vi "ReversedEngineering GetDiagramStateMachineInfo.vi"(1 "Path":path=path "C:/Documents and Settings/MikaelH/My Documents/LabView/StateMachine-JKI/StateMachine3.vi", 2 "StateDiagramReverseOptions":T1={"Clear All Current States"=TRUE, "UseMenuItem"=TRUE, "InsertArrayQueuedElementsVI"="", "Add Actions"=TRUE, "StateDiagramSerachActions"={"Action"=enum."OnlyTheseVIs", "VINames"=[], "LimitActions(VIs)"=0}, "AddCaseCommentsAsActions"=FALSE, "IgnoreStatesNotUsed"=FALSE, "CommentsSerachActions"={"MinimumTextLength"=0, "OnlyTopLeftComment"=FALSE, "CommentPrefix"=""}, "TransitionMode"=enum."Add to current transtion text", "ActionMode"=enum."Add to current action text"}, 5 "error in (no error)":errorcluster) -> (15 "States":T5[](array[typedef]), 19 "error out":errorcluster)   [LabVIEW 2014]
uses:
  <resource>/Framework/Providers/Open_GDS/UML/ReversedEngineering/ReversedEngineering StateMachineStateInfo.ctl
  <resource>/Framework/Providers/Open_GDS/UML/ReversedEngineering/private/ReversedEngineering StateDiagramReverseOptions.ctl
  <resource>/Framework/Providers/Open_GDS/UML/ReversedEngineering/private/ReversedEngineering StateDiagramSerachActions.ctl
  <resource>/Framework/Providers/Open_GDS/UML/ReversedEngineering/ReversedEngineering StateAnalyseVIAction.ctl
  <resource>/Framework/Providers/Open_GDS/UML/ReversedEngineering/private/ReversedEngineering StateDiagramCommentSearchType.ctl
  <resource>/Framework/Providers/Open_GDS/UML/StateReverse_class/StateAction.ctl
  <resource>/Framework/Providers/Open_GDS/UML/ReversedEngineering/ReversedEngineering QueuedStateMachinMemoryAction.ctl
  <resource>/Framework/Providers/Open_GDS/UML/UMLEditor/UMLEditor BusyDialogAction.ctl
  <resource>/Framework/Providers/Open_GDS/ClassProviders/Common/ScriptingFunctions/Scripting.lvclass
  <resource>/Framework/Providers/Open_GDS/UML/StateReverse_class/StateReverse.lvclass
panel:
  out "StateTransitions":cluster{"StateTransitions":string[]}[](array[cluster])
  out "SubViNames":string[](array[string])
  out "Selector Strings":string[](array[string])
  # "C:\\Documents and Settings\\Micke\\Mina dokument\\LabView\\StateMachines\\String1\\StateString1.vi"
  # "C:\\Documents and Settings\\MikaelH\\My Documents\\LabView\\StateMachine-JKI\\StateMachine3.vi"
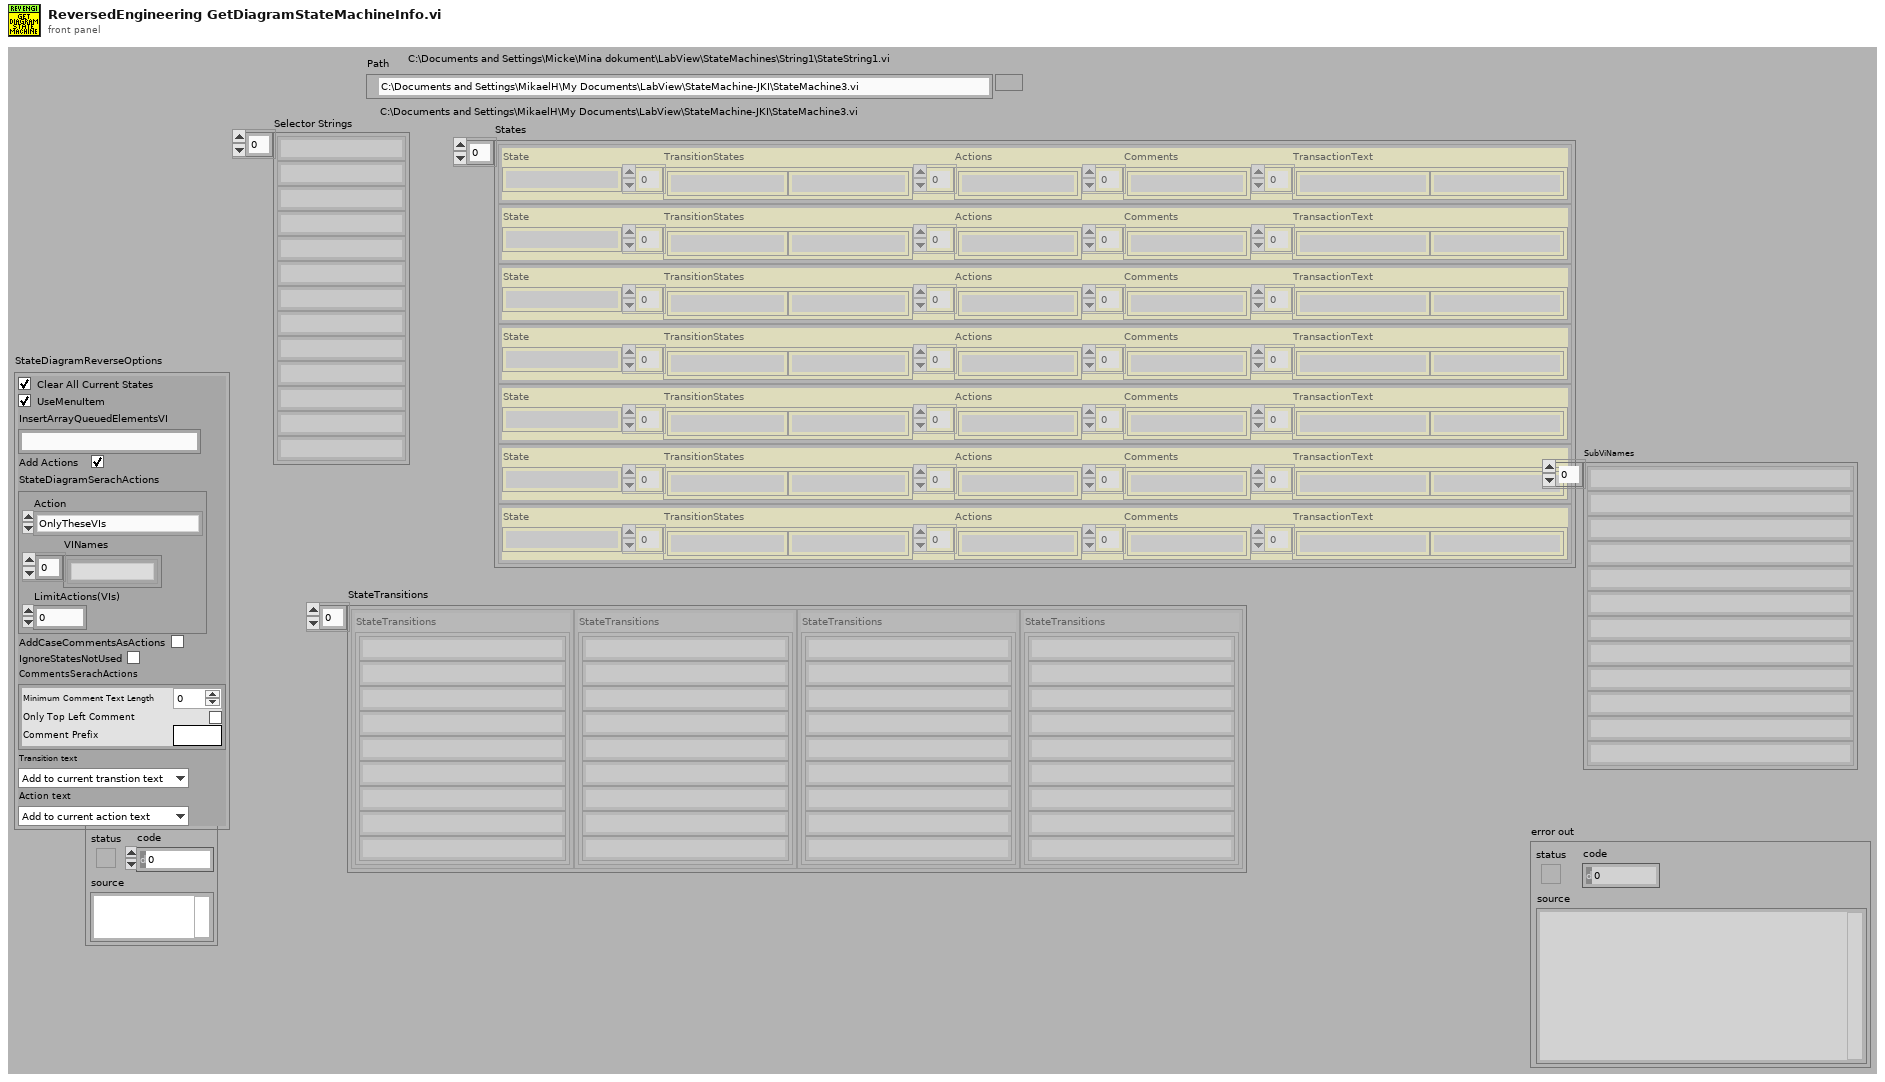
[diagram p1: front panel]
types:
  T1 = typedef "ReversedEngineering StateDiagramReverseOptions.ctl" = cluster{"Clear All Current States":bool, "UseMenuItem":bool, "InsertArrayQueuedElementsVI":string, "Add Actions":bool, "StateDiagramSerachActions":T2, "AddCaseCommentsAsActions":bool, "IgnoreStatesNotUsed":bool, "CommentsSerachActions":T4, "TransitionMode":enum16{"Add to current transtion text", "Replace transition text"}, "ActionMode":enum16{"Add to current action text", "Replace action text"}}
  T2 = typedef "ReversedEngineering StateDiagramSerachActions.ctl" = cluster{"Action":T3, "VINames":string[], "LimitActions(VIs)":i32}
  T3 = typedef "ReversedEngineering StateAnalyseVIAction.ctl" = enum16{"OnlyTheseVIs", "NotTheseVIs"}
  T4 = typedef "ReversedEngineering StateDiagramCommentSearchType.ctl" = cluster{"MinimumTextLength":i32, "OnlyTopLeftComment":bool, "CommentPrefix":string}
  T5 = typedef "ReversedEngineering StateMachineStateInfo.ctl" = cluster{"State":string, "TransitionStates":string[], "Actions":string[], "Comments":string[], "TransactionText":string[]}
  T6 = typedef "Scripting.lvclass/Scripting_PastThroughObjectType.ctl" = cluster{"Object":refnum<vi>, "InsideArray":bool, "PastThroughObjectTypes":T7[], "ObjectType":string, "ObjectData":string}
  T7 = typedef "Scripting_ObjectType.ctl" = cluster{"ObjectType":string, "ObjectName":string, "ObjectTerminalName":string}
  T8 = typedef "StateReverse.lvclass/StateAction.ctl" = enum16{"Normal", "AddInBeggining", "AddInEnd", "AddIfNothingInQueue"}
  T9 = enum16{"NormalSubVis", "LV-Internal VIs", "All VIs", "All Functions"}
  T10 = typedef "ReversedEngineering QueuedStateMachinMemoryAction.ctl" = enum16{"Initialize", "GetInsertQueuedArrayElementsVI", "SetQueuedStateJumps", "GetQueuedStateJumps"}
  T11 = typedef "UMLEditor BusyDialogAction.ctl" = enum16{"Initialize", "Open(VIs)", "Open(i)", "Send_I-Value", "SendStatusMessage", "GetBusyDialogStatus", "Close", "Quit"}
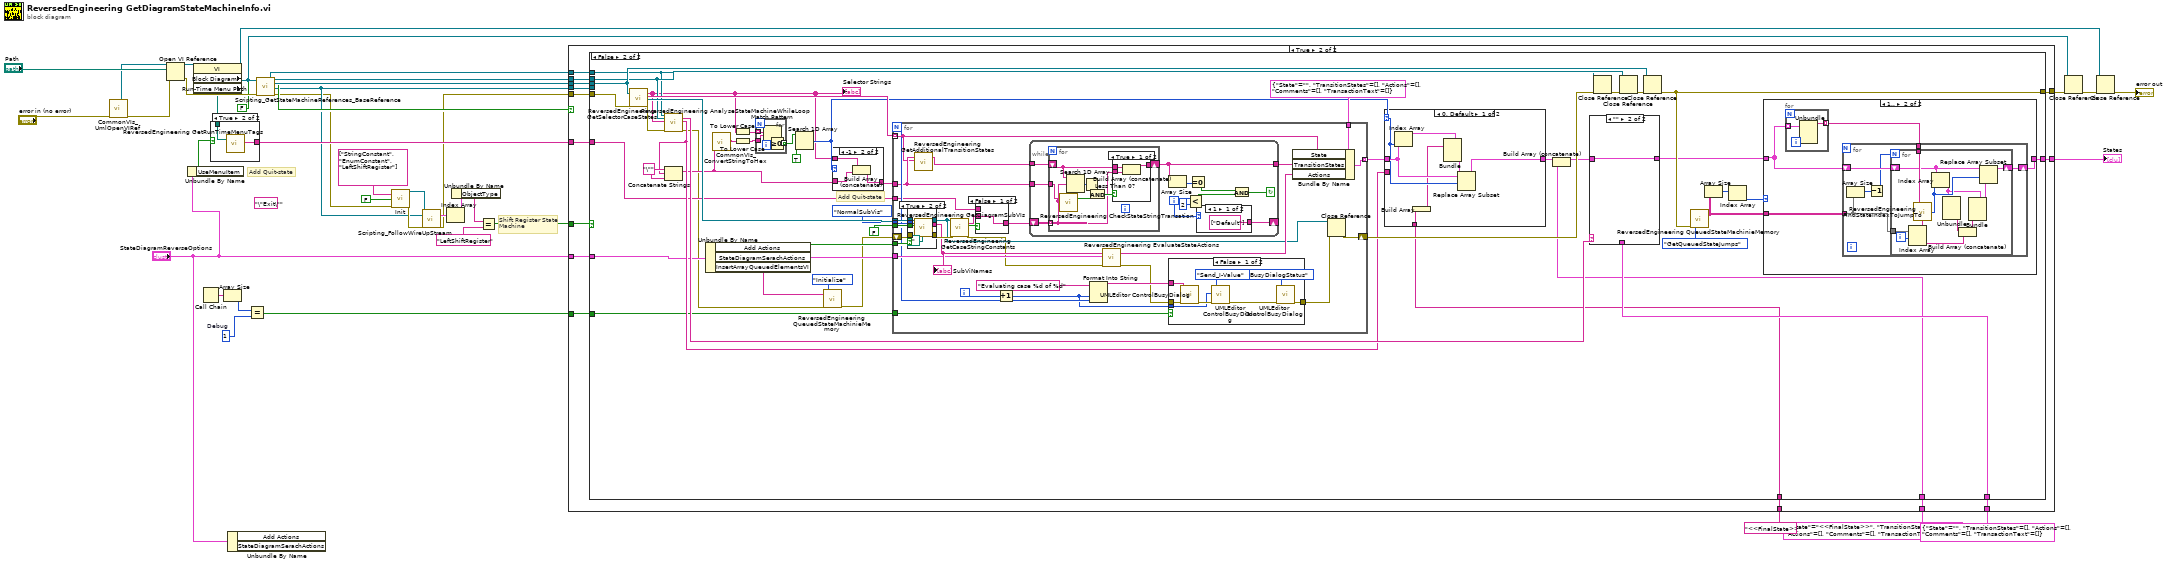
[diagram p0: block diagram]
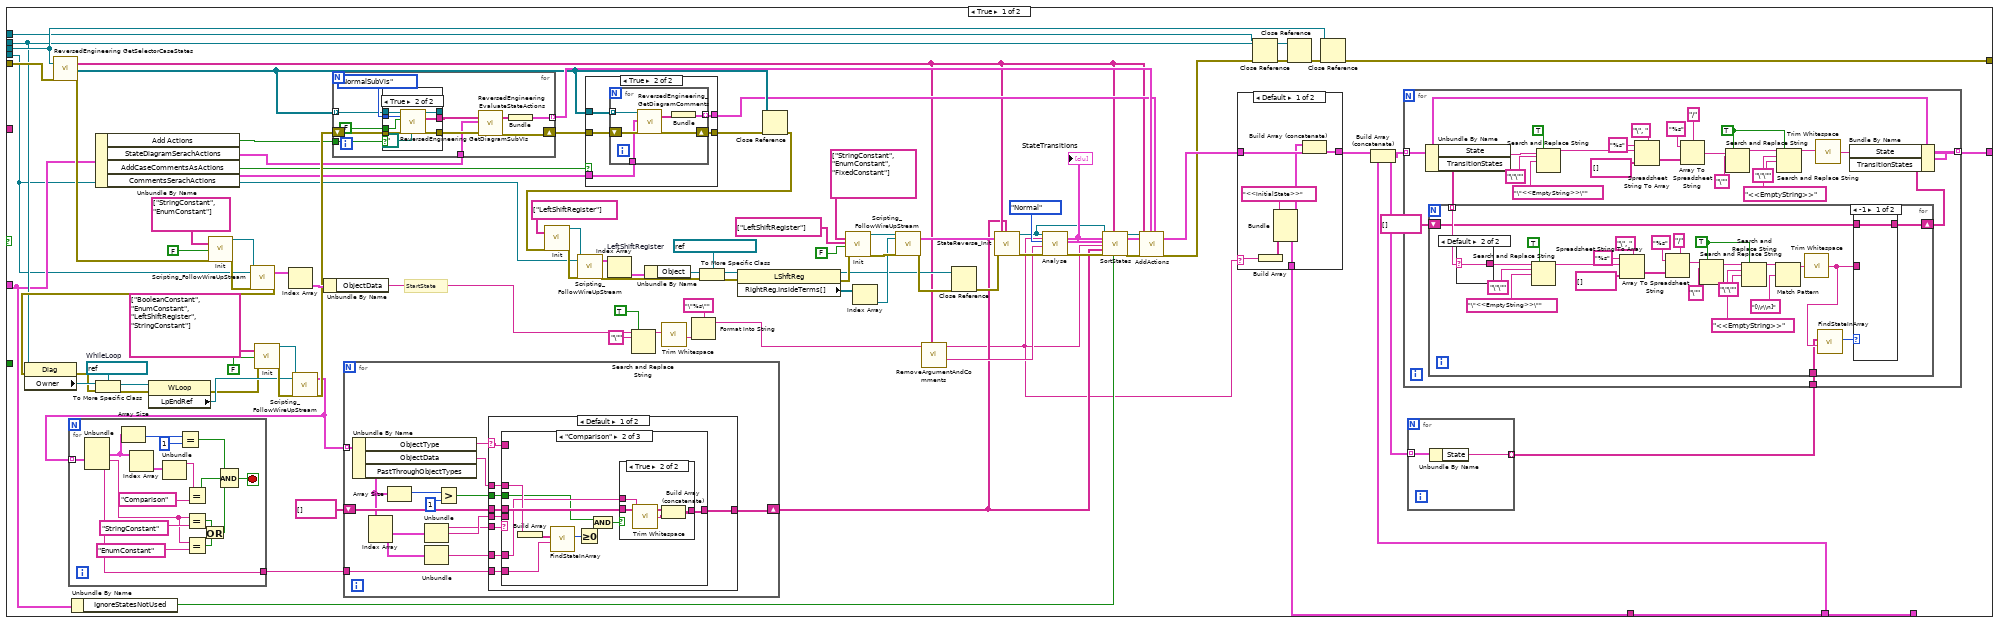
[diagram p4: hidden frame]
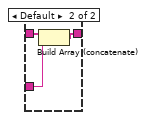
[diagram p7: hidden frame]
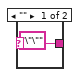
[diagram p8: hidden frame]
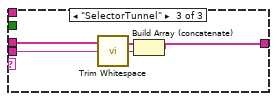
[diagram p11: hidden frame]
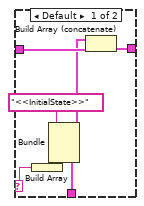
[diagram p15: hidden frame]
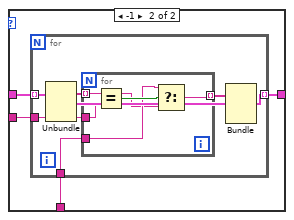
[diagram p16: hidden frame]
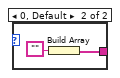
[diagram p18: hidden frame]
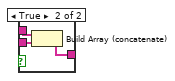
[diagram p20: hidden frame]
diagram:
  w24 = 1  # Debug
  (unwired) "\"Exit\"" ("element")
  # "Shift Register State\nMachine"
  # "Add Quit-state"
  n1 = call <resource>:"CommonVIs_UmlOpenVIRef.vi"("error in"="error in (no error)") -> ("error out"=w2:errorcluster, "AppRefOut"=w1:refnum<vi>)  [unwired: 3 in, 6 out]
  n2 = Open VI Reference(application reference (local)=w1, vi path="Path", error in (no error)=w2) -> (vi reference=w22:refnum<vi>, error out=w39:errorcluster)  [unwired: 3 out]
  n3 = Unbundle By Name("StateDiagramReverseOptions") -> ("UseMenuItem"=w19:bool)
  n4 = property class="VI"(reference=w22) -> (reference out=w32:refnum<vi>, "Block Diagram"=w21:refnum<vi>, "Run-Time Menu Path"=w20:path)  [unwired: 1 in, 1 out]
  n5 = Call Chain() -> (call chain=w26:string[])
  n6 = case shown="True" w19 {
    tunnel: w20 -> [_ w42]
    tunnel: [_ w41] -> w18
    frame False {
    }
    frame True {
      n7 = call <resource>:"ReversedEngineering GetRunTimeMenuTags.vi"("StateMachineCaseSelector"=w42) -> ("ItemTags"=w41:string[])  [unwired: 1 in, 17 out]
    }
  }
  n8 = Array Size(array=w26) -> (size(s)=w25:i32)
  n9 = Unbundle By Name("StateDiagramReverseOptions") -> ()  [unwired: 2 out]
  n10 = Equal?(x=w25, y=w24) -> (x = y?=w23:bool)
  n11 = call <resource>:"Scripting_GetStateMachineReferences_BaseReference.vi"("Diagram"=w21, "WhileLoop(False)"=FALSE, "error in (no error)"=w39) -> ("OutSideWhileLoopDiagram"=w34:refnum<vi>, "StateMachine-WhileLoopDiagram"=w35:refnum<vi>, "StateMachine-CaseSelector"=w38:refnum<vi>, "Found"=w37:bool, "Selector.Outside Terminal"=w12:refnum<vi>, "error out"=w6:errorcluster)  [unwired: 11 in]
  n12 = call <resource>:"Init.vi"("FindAnyOfTheseClassTypes"=string[] ["StringConstant", "EnumConstant", "LeftShiftRegister"], "KeepObjectsOpen(True)"=FALSE, "error in (no error)"=w6) -> ("object out"=w13:refnum<class "Scripting.lvclass">, "error out"=w14:errorcluster)  [unwired: 15 in]
  n13 = call-dynamic "Scripting_FollowWireUpStream.vi"("Scripting in"=w13, "StartTerminalRef"=w12, "error in (no error)"=w14) -> ("FoundItems"=w11:T6[], "error out"=w5:errorcluster)  [unwired: 15 in]
  n14 = Index Array(array=w11) -> (element=w10:T6)  [unwired: 1 in]
  n15 = Unbundle By Name(w10) -> ("ObjectType"=w9:string)
  n16 = Equal?(x=w9, y="LeftShiftRegister" ("StopWhenThisClassTypeReached")) -> (x = y?=w7:bool)
  n17 = case shown="True" w37 {
    tunnel: w38 -> [_ w57]
    tunnel: w5 -> [w43 w50]
    tunnel: [w43 w47] -> w31
    tunnel: [_ w46] -> w36
    tunnel: w35 -> [_ w56]
    tunnel: w34 -> [_ w55]
    tunnel: T5 {"State"="", "TransitionStates"=[], "Actions"=[], "Comments"=[], "TransactionText"=[]} ("State") -> [_ w54]
    tunnel: T5 {"State"="<<FinalState>>", "TransitionStates"=[], "Actions"=[], "Comments"=[], "TransactionText"=[]} ("State") -> [_ w52]
    tunnel: "<<FinalState>>" ("State") -> [_ w53]
    tunnel: "StateDiagramReverseOptions" -> [_ w51]
    tunnel: w23 -> [_ w49]
    tunnel: w18 -> [_ w48]
    tunnel: w12 -> [_ w45]
    tunnel: w7 -> [_ w44]
    frame False {
    }
    frame True {
      n18 = case shown="False" w44 {
        tunnel: w57 -> [w150 w354]
        tunnel: w56 -> [w124 w351]
        tunnel: w55 -> [w148 w350]
        tunnel: w54 -> [w147 w348]
        tunnel: w53 -> [_ w346]
        tunnel: w52 -> [w88 w344]
        tunnel: w51 -> [w73 w339]
        tunnel: w50 -> [w145 w329]
        tunnel: w49 -> [_ w325]
        tunnel: w48 -> [_ w324]
        tunnel: [w144 w319] -> w47
        tunnel: [w90 w314] -> w46
        tunnel: w45 -> [w71 _]
        frame True {
          w118 = refnum<vi> refnum  # LeftShiftRegister
          w143 = refnum<vi> refnum  # WhileLoop
          # "StartState"
          n19 = call <resource>:"ReversedEngineering GetSelectorCaseStates.vi"("StateMachineCaseSelector"=w150, "error out 2"=w145) -> ("SelStrings"=w63:string[], "Frames[]"=w76:refnum<vi>[], "error out"=w126:errorcluster)  [unwired: 2 in, 13 out]
          n20 = Unbundle By Name(w73) -> ("IgnoreStatesNotUsed"=w72:bool)
          n21 = Unbundle By Name(w73) -> ("Add Actions"=w86:bool, "StateDiagramSerachActions"=w85:T2, "AddCaseCommentsAsActions"=w78:bool, "CommentsSerachActions"=w70:T4)
          n22 = call <resource>:"Init.vi"("FindAnyOfTheseClassTypes"=string[] ["StringConstant", "EnumConstant"], "KeepObjectsOpen(True)"=FALSE, "error in (no error)"=w126) -> ("object out"=w131:refnum<class "Scripting.lvclass">, "error out"=w130:errorcluster)  [unwired: 15 in]
          n23 = call-dynamic "Scripting_FollowWireUpStream.vi"("Scripting in"=w131, "StartTerminalRef"=w71, "error in (no error)"=w130) -> ("FoundItems"=w132:T6[], "error out"=w125:errorcluster)  [unwired: 15 in]
          n24 = property class="Diag"(reference=w124, error in=w125) -> (error out=w133:errorcluster, "Owner"=w134:refnum<vi>)  [unwired: 1 out]
          n25 = To More Specific Class(target class=w143, reference=w134, error in=w133) -> (specific class reference=w142:refnum<vi>, error out=w137:errorcluster)
          n26 = property class="WLoop"(reference=w142, error in=w137) -> (error out=w138:errorcluster, "LpEndRef"=w139:refnum<vi>)  [unwired: 1 out]
          n27 = call <resource>:"Init.vi"("FindAnyOfTheseClassTypes"=string[] ["BooleanConstant", "EnumConstant", "LeftShiftRegister", "StringConstant"], "KeepObjectsOpen(True)"=FALSE, "error in (no error)"=w138) -> ("object out"=w140:refnum<class "Scripting.lvclass">, "error out"=w141:errorcluster)  [unwired: 15 in]
          n28 = Index Array(array=w132) -> (element=w127:T6)  [unwired: 1 in]
          n29 = call-dynamic "Scripting_FollowWireUpStream.vi"("Scripting in"=w140, "StartTerminalRef"=w139, "error in (no error)"=w141) -> ("FoundItems"=w59:T6[], "error out"=w87:errorcluster)  [unwired: 15 in]
          n30 = for {
            tunnel: w59 -> [w167] mode=indexing
            tunnel: [w151] -> w58
            stop <- w152 stop-if-true
            n31 = Unbundle(w167) -> ("PastThroughObjectTypes"=w163:T7[], "ObjectType"=w159:string, "ObjectData"=w151:string)  [unwired: 2 out]
            n32 = Array Size(array=w163) -> (size(s)=w162:i32)
            n33 = Index Array(array=w163) -> (element=w164:T7)  [unwired: 1 in]
            n34 = Unbundle(w164) -> ("ObjectType"=w166:string)  [unwired: 2 out]
            n35 = Equal?(x=w162, y=1) -> (x = y?=w155:bool)
            n36 = Equal?(x=w166, y="Comparison") -> (x = y?=w154:bool)
            n37 = Equal?(x=w159, y="StringConstant" ("StopWhenThisClassTypeReached")) -> (x = y?=w157:bool)
            n38 = Equal?(x=w159, y="EnumConstant" ("StopWhenThisClassTypeReached")) -> (x = y?=w156:bool)
            n39 = Or(x=w157, y=w156) -> (x .or. y?=w153:bool)
            n40 = Compound Arithmetic op=AND(w155, w154, w153) -> (w152:bool)
          }
          n41 = Unbundle By Name(w127) -> ("ObjectData"=w91:string)
          n42 = for {
            tunnel: w86 -> [w192]
            shift-right: [w187] -> w79
            shift-left: w87 -> [w190]
            tunnel: w85 -> [w185]
            tunnel: w76 -> [w184] mode=indexing
            tunnel: [w182] -> w80 mode=indexing
            n43 = case shown="True" w192 {
              tunnel: [w193 w202] -> _
              tunnel: w190 -> [w194 w201]
              tunnel: [w194 w200] -> w191
              tunnel: T9."NormalSubVis" ("SubVIsOptions(NormalSubVis)") -> [_ w199]
              tunnel: [_ w198] -> w186
              tunnel: FALSE ("RecrsiveSearchInNormalSubVIs(False)") -> [_ w197]
              tunnel: w184 -> [w193 w196]
              frame False {
              }
              frame True {
                n44 = call <resource>:"ReversedEngineering GetDiagramSubVIs.vi"("Diagram"=w196, "SubVIsOptions(NormalSubVis)"=w199, "RecrsiveSearchInNormalSubVIs(False)"=w197, "error in (no error)"=w201, "PathToDebugVI(OnlyUsedForRecursivVitFiles)"=path "") -> ("DiagramOut"=w202:refnum<vi>, "SubViNames"=w198:string[], "error out"=w200:errorcluster)  [unwired: 12 out]
              }
            }
            n45 = call <resource>:"ReversedEngineering EvaluateStateActions.vi"("SubViNames"=w186, "StateDiagramSerachActions"=w185, "error in"=w191) -> ("StateActions"=w183:string[], "error out"=w187:errorcluster)  [unwired: 15 out]
            n46 = Bundle("StateActions"=w183) -> (w182:cluster{"StateActions":string[]})  [unwired: 1 in]
          }
          n47 = for {
            tunnel: w59 -> [w274] mode=indexing
            shift-right: [w271] -> w62
            shift-left: string[] [] -> [w272]
            tunnel: w58 -> [w264]
            n48 = Unbundle By Name(w274) -> ("ObjectType"=w273:string, "ObjectData"=w268:string, "PastThroughObjectTypes"=w261:T7[])
            n49 = Index Array(array=w261) -> (element #1=w267:T7, element #2=w266:T7)  [unwired: 2 in]
            n50 = Array Size(array=w261) -> (size(s)=w263:i32)
            n51 = Unbundle(w267) -> ("ObjectType"=w269:string, "ObjectName"=w270:string)  [unwired: 1 out]
            n52 = Unbundle(w266) -> ("ObjectName"=w265:string)  [unwired: 2 out]
            n53 = Greater?(x=w263, y=1) -> (0:w260:bool)
            n54 = case shown="Default" w273 {
              selector: w273 -> [w279 _]
              tunnel: w272 -> [w283 w304]
              tunnel: [w282 w304] -> w271
              tunnel: w270 -> [w281 _]
              tunnel: w269 -> [w280 _]
              tunnel: w268 -> [w278 _]
              tunnel: w265 -> [w277 _]
              tunnel: w264 -> [w276 _]
              tunnel: w260 -> [w275 _]
              frame Default {
                n55 = case shown="\"Comparison\"" w280 {
                  tunnel: w283 -> [w284 w294 w303]
                  tunnel: [w284 w293 w302] -> w282
                  tunnel: w281 -> [_ _ w301]
                  tunnel: w279 -> [_ _ _]
                  tunnel: w278 -> [_ w289 _]
                  tunnel: w277 -> [_ w288 _]
                  tunnel: w276 -> [_ w290 _]
                  tunnel: w275 -> [_ w285 _]
                  frame Default {
                  }
                  frame "Comparison" {
                    n56 = Build Array(w289) -> (w291:string[])
                    n57 = call <resource>:"FindStateInArray.vi"("TransactionState"=w290, "AllCaseStates"=w291) -> ("index of element"=w292:i32)  [unwired: 7 in, 2 out]
                    n58 = Greater Or Equal To 0?(x=w292) -> (x >= 0?=w287:bool)
                    n59 = And(x=w285, y=w287) -> (x .and. y?=w286:bool)
                    n60 = case shown="True" w286 {
                      tunnel: w294 -> [w295 w298]
                      tunnel: [w295 w297] -> w293
                      tunnel: w288 -> [_ w296]
                      frame False {
                      }
                      frame True {
                        n61 = call <vilib>:"Trim Whitespace.vi"("string"=w296) -> ("trimmed string"=w299:string)  [unwired: 1 in]
                        n62 = Build Array (concatenate)(w298, w299) -> (w297:string[])
                      }
                    }
                  }
                  frame "SelectorTunnel" {
                    n63 = call <vilib>:"Trim Whitespace.vi"("string"=w301) -> ("trimmed string"=w300:string)  [unwired: 1 in]
                    n64 = Build Array (concatenate)(w303, w300) -> (w302:string[])
                  }
                }
              }
              frame "UseDefault" {
              }
            }
          }
          n65 = case shown="True" w78 {
            tunnel: w79 -> [w170 w175]
            tunnel: w76 -> [_ w174]
            tunnel: [w170 w173] -> w77
            tunnel: [_ w172] -> w75
            tunnel: w70 -> [_ w171]
            frame False {
            }
            frame True {
              n66 = for {
                tunnel: w174 -> [w180] mode=indexing
                shift-right: [w179] -> w173
                shift-left: w175 -> [w181]
                tunnel: [w177] -> w172 mode=indexing
                tunnel: w171 -> [w176]
                n67 = call <resource>:"ReversedEngineering_GetDiagramComments.vi"("Diagram"=w180, "CommentsSerachActions"=w176, "error in"=w181) -> ("Comments"=w178:string[], "error out"=w179:errorcluster)  [unwired: 15 in]
                n68 = Bundle("Comments"=w178) -> (w177:cluster{"Comments":string[]})  [unwired: 1 in]
              }
            }
          }
          n69 = Search and Replace String(replace all?=TRUE ("replace all? (F)"), input string=w91, search string="\"") -> (result string=w94:string)  [unwired: 5 in, 3 out]
          n70 = call <vilib>:"Trim Whitespace.vi"("string"=w94) -> ("trimmed string"=w92:string)  [unwired: 1 in]
          n71 = Format Into String(format string="\"%s\"", w92) -> (resulting string=w65:string)  [unwired: 2 in, 1 out]
          n72 = Close Reference(reference=w76, error in (no error)=w77) -> (error out=w74:errorcluster)
          n73 = call <resource>:"Init.vi"("FindAnyOfTheseClassTypes"=string[] ["LeftShiftRegister"], "error in (no error)"=w74) -> ("object out"=w122:refnum<class "Scripting.lvclass">, "error out"=w123:errorcluster)  [unwired: 16 in]
          n74 = call-dynamic "Scripting_FollowWireUpStream.vi"("Scripting in"=w122, "StartTerminalRef"=w71, "error in (no error)"=w123) -> ("FoundItems"=w121:T6[], "error out"=w117:errorcluster)  [unwired: 15 in]
          n75 = Index Array(array=w121) -> (element=w120:T6)  [unwired: 1 in]
          n76 = Unbundle By Name(w120) -> ("Object"=w119:refnum<vi>)
          n77 = To More Specific Class(target class=w118, reference=w119, error in=w117) -> (specific class reference=w116:refnum<vi>, error out=w115:errorcluster)
          n78 = property class="LShftReg"(reference=w116, error in=w115) -> (reference out=w104:refnum<vi>, error out=w109:errorcluster, "RightReg.InsideTerms[]"=w114:refnum<vi>[])
          n79 = call <resource>:"Init.vi"("FindAnyOfTheseClassTypes"=string[] ["StringConstant", "EnumConstant", "FixedConstant"], "StopWhenAnyOfTheseClassTypesAreReached"=string[] ["LeftShiftRegister"] ("FindAnyOfTheseClassTypes"), "KeepObjectsOpen(True)"=FALSE, "error in (no error)"=w109) -> ("object out"=w111:refnum<class "Scripting.lvclass">, "error out"=w113:errorcluster)  [unwired: 14 in]
          n80 = Index Array(array=w114) -> (element=w110:refnum<vi>)  [unwired: 1 in]
          n81 = call-dynamic "Scripting_FollowWireUpStream.vi"("Scripting in"=w111, "StartTerminalRef"=w110, "error in (no error)"=w113) -> ("FoundItems"=w100:T6[], "error out"=w105:errorcluster)  [unwired: 15 in]
          n82 = call <resource>:"RemoveArgumentAndComments.vi"("AllCaseStates"=w63, "TransactionStateIn"=w65) -> ("Comment"=w64:string, "TransactionStateOut"=w61:string)  [unwired: 7 in, 1 out]
          n83 = Close Reference(reference=w104, error in (no error)=w105) -> (error out=w101:errorcluster)
          n84 = call <resource>:"StateReverse_Init.vi"("StatesData"=w100, "error in (no error)"=w101, "StateStrings"=w63, "ExitStates"=w62) -> ("object out"=w67:refnum<class "StateReverse.lvclass">, "error out"=w103:errorcluster)  [unwired: 14 in]
          n85 = call-dynamic "Analyse.vi"("object in"=w67, "NextState"=w61, "StateAction"=StateAction."Normal", "NextStateComments"=w64, "error in (no error)"=w103) -> ("StateTransitions"=w98:cluster{"StateTransitions":string[]}[], "CommentsTransitions"=w60:cluster{"StateTransitions":string[]}[], "error out"=w97:errorcluster)  [unwired: 12 in]
          "StateTransitions" <- w98
          n86 = call <resource>:"SortStates.vi"("object in"=w67, "StateTransitions"=w98, "CommentsTransitions"=w60, "StartState"=w61, "ExitStates"=w62, "error in (no error)"=w97, "StateStrings"=w63, "RemoveStatesNotInUse(True)"=w72) -> ("object out"=w66:refnum<class "StateReverse.lvclass">, "States"=w84:T5[], "error out"=w83:errorcluster)  [unwired: 9 in]
          n87 = call <resource>:"AddActions.vi"("object in"=w66, "StatesIn"=w84, "error in (no error)"=w83, "StateStrings"=w63, "StateActions"=w80, "StateComments"=w75) -> ("States"=w82:T5[], "error out"=w81:errorcluster)  [unwired: 11 in, 1 out]
          n88 = case shown="Default" w61 {
            selector: w61 -> [w307 _]
            tunnel: w82 -> [w311 w312]
            tunnel: [w310 w312] -> w89
            tunnel: w147 -> [w309 _]
            frame Default {
              n89 = Build Array(w307) -> (w306:string[])
              n90 = Bundle(cluster=w309, "State"="<<InitialState>>", "TransitionStates"=w306) -> (w305:T5)  [unwired: 3 out]
              n91 = Build Array (concatenate)(w305, w311) -> (w310:T5[])
            }
            frame "" {
            }
          }
          n92 = Close Reference(reference=w148, error in (no error)=w81) -> (error out=w149:errorcluster)
          n93 = Close Reference(reference=w124, error in (no error)=w149) -> (error out=w146:errorcluster)
          n94 = Close Reference(reference=w150, error in (no error)=w146) -> (error out=w144:errorcluster)
          n95 = Build Array (concatenate)(w89, w88) -> (w69:T5[])
          n96 = for {
            tunnel: w69 -> [w169] mode=indexing
            tunnel: [w168] -> w68 mode=indexing
            n97 = Unbundle By Name(w169) -> ("State"=w168:string)
          }
          n98 = for {
            tunnel: w69 -> [w219] mode=indexing
            tunnel: [w217] -> w90 mode=indexing
            tunnel: w68 -> [w203]
            w210 = TRUE ("replace all? (F)")
            n99 = Unbundle By Name(w219) -> ("State"=w214:string, "TransitionStates"=w218:string[])
            n100 = for {
              tunnel: w218 -> [w244] mode=indexing
              shift-right: [w232] -> w205
              shift-left: string[] [] -> [w231]
              tunnel: w203 -> [w228]
              w233 = TRUE ("replace all? (F)")
              n101 = case shown="Default" w244 {
                selector: w244 -> [_ w259]
                tunnel: ["\"\"" ("delimiter (Tab)") w259] -> w253
                frame "" {
                }
                frame Default {
                }
              }
              n102 = Search and Replace String(replace all?=TRUE ("replace all? (F)"), input string=w253, search string="\"\"" ("delimiter (Tab)"), replace string="\"<<EmptyString>>\"" ("delimiter (Tab)")) -> (result string=w238:string)  [unwired: 4 in, 3 out]
              n103 = Spreadsheet String To Array(delimiter (Tab)="\", ", format string="%s", spreadsheet string=w238, array type (2D Dbl)=string[] []) -> (array=w242:string[])
              n104 = Array To Spreadsheet String(delimiter (Tab)="/", array=w242, 3:"%s" ("format string")) -> (spreadsheet string=w234:string)
              n105 = Search and Replace String(replace all?=w233, input string=w234, search string="\"" ("delimiter (Tab)")) -> (result string=w235:string)  [unwired: 5 in, 3 out]
              n106 = Search and Replace String(replace all?=w233, input string=w235, search string="<<EmptyString>>" ("delimiter (Tab)"), replace string="\"\"" ("delimiter (Tab)")) -> (result string=w250:string)  [unwired: 4 in, 3 out]
              n107 = Match Pattern(string=w250, regular expression="[\\r\\n]") -> (before substring=w252:string)  [unwired: 1 in, 3 out]
              n108 = call <vilib>:"Trim Whitespace.vi"("string"=w252) -> ("trimmed string"=w230:string)  [unwired: 1 in]
              n109 = call <resource>:"FindStateInArray.vi"("TransactionState"=w230, "AllCaseStates"=w228) -> ("index of element"=w229:i32)  [unwired: 7 in, 2 out]
              n110 = case shown="-1" w229 {
                tunnel: [w254 w257] -> w232
                tunnel: w230 -> [_ w256]
                tunnel: w231 -> [w254 w255]
                frame -1 {
                }
                frame Default {
                  n111 = Build Array (concatenate)(w255, w256) -> (w257:string[])
                }
              }
            }
            n112 = Search and Replace String(replace all?=TRUE ("replace all? (F)"), input string=w214, search string="\"\"" ("delimiter (Tab)"), replace string="\"<<EmptyString>>\"" ("delimiter (Tab)")) -> (result string=w213:string)  [unwired: 4 in, 3 out]
            n113 = Spreadsheet String To Array(delimiter (Tab)="\", ", format string="%s", spreadsheet string=w213, array type (2D Dbl)=string[] []) -> (array=w224:string[])
            n114 = Array To Spreadsheet String(delimiter (Tab)="/", array=w224, 3:"%s" ("format string")) -> (spreadsheet string=w221:string)
            n115 = Search and Replace String(replace all?=w210, input string=w221, search string="\"" ("delimiter (Tab)")) -> (result string=w211:string)  [unwired: 5 in, 3 out]
            n116 = Search and Replace String(replace all?=w210, input string=w211, search string="<<EmptyString>>" ("delimiter (Tab)"), replace string="\"\"" ("delimiter (Tab)")) -> (result string=w207:string)  [unwired: 4 in, 3 out]
            n117 = call <vilib>:"Trim Whitespace.vi"("string"=w207) -> ("trimmed string"=w206:string)  [unwired: 1 in]
            n118 = Bundle By Name(cluster=w219, "State"=w206, "TransitionStates"=w205) -> (w217:T5)
          }
        }
        frame False {
          w347 = "\"" ("string")
          # "Add Quit-state"
          n119 = call <resource>:"ReversedEngineering GetSelectorCaseStates.vi"("StateMachineCaseSelector"=w354, "error out 2"=w329) -> ("SelStrings"=w328:string[], "StateStrings"=w356:string[], "Frames[]"=w355:refnum<vi>[], "error out"=w330:errorcluster)  [unwired: 2 in, 12 out]
          "Selector Strings" <- w328
          n120 = call <resource>:"ReversedEngineering AnalyseStateMachineWhileLoop.vi"("OutSideWhileLoop"=w350, "StateWhileLoop"=w351, "SelStrings"=w328, "error in"=w330) -> ("InitialState"=w349:string, "FinallState"=w343:string, "error out"=w321:errorcluster)  [unwired: 13 out]
          n121 = Concatenate Strings(w347, w343, w347) -> (w335:string)
          n122 = Unbundle By Name(w339) -> ("Add Actions"=w332:bool, "StateDiagramSerachActions"=w331:T2, "InsertArrayQueuedElementsVI"=w322:string)
          n123 = call <resource>:"CommonVIs_ConvertStringToHex.vi"("inputString"=w335) -> ("outputString"=w336:string)  [unwired: 1 in, 17 out]
          n124 = To Lower Case(string=w328) -> (all lower case string=w327:string[])
          n125 = To Lower Case(string=w336) -> (all lower case string=w326:string)
          n126 = for {
            tunnel: w327 -> [w388] mode=indexing
            tunnel: [w386] -> w338 mode=indexing
            tunnel: w326 -> [w385]
            n127 = Match Pattern(string=w388, regular expression=w385) -> (offset past match=w387:i32)  [unwired: 4 out]
            n128 = Greater Or Equal To 0?(x=w387) -> (x >= 0?=w386:bool)
          }
          n129 = Search 1D Array(1D array=w338, element=TRUE) -> (index of element=w334:i32)  [unwired: 1 out]
          n130 = call <resource>:"ReversedEngineering QueuedStateMachinieMemory.vi"("VIName"=w322, "error in (no error)"=w321, "Action(GetInsertQueuedArrayElementsVI)"=ReversedEngineering_QueuedStateMachinMemoryAction."Initialize" ("Action(GetInsertQueuedArrayElements)")) -> ("error out"=w320:errorcluster)  [unwired: 1 in, 15 out]
          n131 = case shown="-1" w334 {
            tunnel: [w419 w421] -> w358
            tunnel: w335 -> [_ w422]
            tunnel: w328 -> [w419 w420]
            frame 0, Default {
            }
            frame -1 {
              n132 = Build Array (concatenate)(w420, w422) -> (w421:string[])
            }
          }
          n133 = for {
            N -> [w436]
            shift-right: [w428] -> w353
            shift-left: w320 -> [w448]
            tunnel: w358 -> [w432]
            tunnel: T5 {"State"="", "TransitionStates"=[], "Actions"=[], "Comments"=[], "TransactionText"=[]} ("State") -> [w452]
            tunnel: [w450] -> w357 mode=indexing
            tunnel: w356 -> [w431] mode=indexing
            tunnel: w355 -> [w449] mode=indexing
            tunnel: T9."NormalSubVis" ("SubVIsOptions(NormalSubVis)") -> [w446]
            tunnel: FALSE ("RecrsiveSearchInNormalSubVIs(False)") -> [w445]
            tunnel: w331 -> [w442]
            tunnel: w332 -> [w441]
            tunnel: w325 -> [w427]
            tunnel: w324 -> [w424]
            i -> [w437]
            n134 = case shown="True" w441 {
              tunnel: [w493 w501] -> w440
              tunnel: w449 -> [w493 w500]
              tunnel: w448 -> [w492 w499]
              tunnel: [w492 w498] -> w447
              tunnel: w446 -> [_ w497]
              tunnel: w445 -> [_ w496]
              tunnel: [_ w495] -> w444
              frame False {
              }
              frame True {
                n135 = call <resource>:"ReversedEngineering GetDiagramSubVIs.vi"("Diagram"=w500, "SubVIsOptions(NormalSubVis)"=w497, "RecrsiveSearchInNormalSubVIs(False)"=w496, "error in (no error)"=w499, "PathToDebugVI(OnlyUsedForRecursivVitFiles)"=path "") -> ("DiagramOut"=w501:refnum<vi>, "SubViNames"=w495:string[], "error out"=w498:errorcluster)  [unwired: 12 out]
              }
            }
            "SubViNames" <- w444
            n136 = call <resource>:"ReversedEngineering GetAdditionalTransitionStates.vi"("SelStrings"=w432, "StringConstant"=w431) -> ("AdditionalTransitionStates"=w430:string[])  [unwired: 17 out]
            n137 = call <resource>:"ReversedEngineering GetCaseStringConstants.vi"("Diagram"=w440, "error in (no error)"=w447) -> ("StringConstants"=w425:string[], "EventStructureUsed"=w426:bool, "error out"=w434:errorcluster)  [unwired: 15 out]
            n138 = case shown="False" w426 {
              tunnel: w425 -> [w479 w481]
              tunnel: [w479 w482] -> w423
              tunnel: w424 -> [_ w480]
              frame False {
              }
              frame True {
                n139 = Build Array (concatenate)(w480, w481) -> (w482:string[])
              }
            }
            n140 = Increment(x=w437) -> (x+1=w435:i32)
            n141 = while {
              tunnel: [w461] -> w451
              tunnel: w432 -> [w463]
              tunnel: w430 -> [w462]
              shift-right: [w455] -> _
              shift-left: w423 -> [w460]
              i -> [w453]
              stop <- w456 continue-if-true
              n142 = for {
                tunnel: w460 -> [w468] mode=indexing
                tunnel: w463 -> [w469]
                shift-right: [w474] -> w461
                shift-left: w462 -> [w473]
                n143 = call <resource>:"ReversedEngineering CheckStateStringTransation.vi"("SelStrings"=w469, "StringConstant"=w468) -> ("Found"=w467:bool)  [unwired: 2 in, 15 out]
                n144 = Search 1D Array(1D array=w473, element=w468) -> (index of element=w471:i32)  [unwired: 1 out]
                n145 = Less Than 0?(x=w471) -> (x < 0?=w470:bool)
                n146 = And(x=w470, y=w467) -> (x .and. y?=w472:bool)
                n147 = case shown="True" w472 {
                  tunnel: w468 -> [w477 _]
                  tunnel: w473 -> [w476 w478]
                  tunnel: [w475 w478] -> w474
                  frame True {
                    n148 = Build Array (concatenate)(w476, w477) -> (w475:string[])
                  }
                  frame False {
                  }
                }
              }
              n149 = Array Size(array=w461) -> (size(s)=w459:i32)
              n150 = Less?(x=w453, y=2) -> (x < y?=w457:bool)
              n151 = Equal To 0?(x=w459) -> (x = 0?=w458:bool)
              n152 = case shown="1" w453 {
                tunnel: [string[] ["Default"] ("StringConstants") w465] -> w455
                frame 1 {
                }
                frame 0, Default {
                  n153 = Build Array("") -> (w465:string[])
                }
              }
              n154 = And(x=w458, y=w457) -> (x .and. y?=w456:bool)
            }
            n155 = Format Into String(format string="Evaluating case %d of %d", w435, w436) -> (resulting string=w438:string)  [unwired: 2 in, 1 out]
            n156 = call <resource>:"ReversedEngineering EvaluateStateActions.vi"("SubViNames"=w444, "StateDiagramSerachActions"=w442, "error in"=w434) -> ("StateActions"=w443:string[], "error out"=w433:errorcluster)  [unwired: 15 out]
            n157 = case shown="False" w427 {
              tunnel: w438 -> [w490 _]
              tunnel: w435 -> [w487 _]
              tunnel: w433 -> [w485 w491]
              tunnel: [w483 w491] -> w429
              frame False {
                n158 = call <resource>:"UMLEditor ControlBusyDialog.vi"("Title/StatusText"=w490, "error in (no error)"=w485) -> ("error out"=w489:errorcluster)  [unwired: 2 in, 15 out]
                n159 = call <resource>:"UMLEditor ControlBusyDialog.vi"("I-Value"=w487, "error in (no error)"=w489, "Action(SendStatusMessage)"=UMLEditor_BusyDialogAction."Send_I-Value") -> ("error out"=w484:errorcluster)  [unwired: 1 in, 15 out]
                n160 = call <resource>:"UMLEditor ControlBusyDialog.vi"("error in (no error)"=w484, "Action(SendStatusMessage)"=UMLEditor_BusyDialogAction."GetBusyDialogStatus") -> ("error out"=w483:errorcluster)  [unwired: 2 in, 15 out]
              }
              frame True {
              }
            }
            n161 = Bundle By Name(cluster=w452, "State"=w431, "TransitionStates"=w451, "Actions"=w443) -> (w450:T5)
            n162 = Close Reference(reference=w440, error in (no error)=w429) -> (error out=w428:errorcluster)
          }
          n163 = case shown="0, Default" w334 {
            selector: w334 -> [w401 _]
            tunnel: w357 -> [w402 w407]
            tunnel: [w399 w406] -> w345
            tunnel: w346 -> [w398 w405]
            tunnel: w343 -> [_ w404]
            frame 0, Default {
              n164 = Index Array(array=w402, index=w401) -> (element=w403:T5)
              n165 = Build Array(w398) -> (w397:string[])
              n166 = Bundle(cluster=w403, "TransitionStates"=w397) -> (w400:T5)  [unwired: 4 out]
              n167 = Replace Array Subset(array=w402, new element=w400, index=w401) -> (w399:T5[])
            }
            frame -1 {
              n168 = for {
                tunnel: w407 -> [w412] mode=indexing
                tunnel: [w411] -> w406 mode=indexing
                tunnel: w405 -> [w409]
                tunnel: w404 -> [w408]
                n169 = Unbundle(w412) -> ("TransitionStates"=w413:string[])  [unwired: 4 out]
                n170 = for {
                  tunnel: w413 -> [w415] mode=indexing
                  tunnel: [w416] -> w410 mode=indexing
                  tunnel: w409 -> [w417]
                  tunnel: w408 -> [w414]
                  n171 = Equal?(x=w415, y=w414) -> (x = y?=w418:bool)
                  n172 = Select(t=w417, s=w418, f=w415) -> (s? t:f=w416:string)
                }
                n173 = Bundle(cluster=w412, "TransitionStates"=w410) -> (w411:T5)  [unwired: 4 out]
              }
            }
          }
          n174 = Build Array (concatenate)(w345, w344) -> (w342:T5[])
          n175 = case shown="\"\"" w349 {
            selector: w349 -> [w391 _]
            tunnel: w342 -> [w395 w396]
            tunnel: [w394 w396] -> w315
            tunnel: w348 -> [w393 _]
            frame Default {
              n176 = Build Array(w391) -> (w390:string[])
              n177 = Bundle(cluster=w393, "State"="<<InitialState>>", "TransitionStates"=w390) -> (w389:T5)  [unwired: 3 out]
              n178 = Build Array (concatenate)(w389, w395) -> (w394:T5[])
            }
            frame "" {
            }
          }
          n179 = Close Reference(reference=w350, error in (no error)=w353) -> (error out=w352:errorcluster)
          n180 = Close Reference(reference=w351, error in (no error)=w352) -> (error out=w333:errorcluster)
          n181 = Close Reference(reference=w354, error in (no error)=w333) -> (error out=w319:errorcluster)
          n182 = call <resource>:"ReversedEngineering QueuedStateMachinieMemory.vi"("error in (no error)"=w319, "Action(GetInsertQueuedArrayElementsVI)"=ReversedEngineering_QueuedStateMachinMemoryAction."GetQueuedStateJumps") -> ("StateJumpsOut"=w313:string[][])  [unwired: 2 in, 15 out]
          n183 = Array Size(array=w313) -> (size(s)=w317:i32[])
          n184 = Index Array(array=w317) -> (element=w316:i32)  [unwired: 1 in]
          n185 = case shown="1.." w316 {
            tunnel: w315 -> [w360 w363]
            tunnel: [w360 w361] -> w314
            tunnel: w313 -> [_ w364]
            frame 0, Default {
            }
            frame 1.. {
              n186 = for {
                tunnel: w363 -> [w384] mode=indexing
                tunnel: [w383] -> w362 mode=indexing
                n187 = Unbundle(w384) -> ("State"=w383:string)  [unwired: 4 out]
              }
              n188 = for {
                tunnel: w364 -> [w366] mode=indexing
                shift-right: [w365] -> w361
                shift-left: w363 -> [w369]
                tunnel: w362 -> [w367]
                n189 = Array Size(array=w366) -> (size(s)=w370:i32)
                n190 = Decrement(x=w370) -> (x-1=w368:i32)
                n191 = for {
                  N: w368 -> [_]
                  shift-right: [w380] -> w365
                  shift-left: w369 -> [w381]
                  tunnel: w367 -> [w382]
                  tunnel: w366 -> [w374]
                  i -> [w373]
                  n192 = Index Array(array=w374, index #1=w373) -> (element #1=w372:string, element #2=w371:string)  [unwired: 1 in]
                  n193 = call <resource>:"ReversedEngineering FindStateIndexToJumpTo.vi"("String"=w372, "Array"=w382) -> ("index of element"=w379:i32)
                  n194 = Index Array(array=w381, index=w379) -> (element=w378:T5)
                  n195 = Unbundle(w378) -> ("TransitionStates"=w376:string[])  [unwired: 4 out]
                  n196 = Build Array (concatenate)(w376, w371) -> (w375:string[])
                  n197 = Bundle(cluster=w378, "TransitionStates"=w375) -> (w377:T5)  [unwired: 4 out]
                  n198 = Replace Array Subset(array=w381, new element=w377, index=w379) -> (w380:T5[])
                }
              }
            }
          }
        }
      }
    }
  }
  "States" <- w36
  n199 = Close Reference(reference=w21, error in (no error)=w31) -> (error out=w30:errorcluster)
  n200 = Close Reference(reference=w32, error in (no error)=w30) -> (error out=→"error out":errorcluster)
